vi "Init Sync Box.vi"(8 "error in (no error)":errorcluster, 11 "Channel in":refnum<class "Channel.lvclass">) -> (0 "error out":errorcluster, 3 "Channel out":refnum<class "Channel.lvclass">)   [LabVIEW 2018, in "Channel.lvclass"]
uses:
  Channel.lvclass
  Sync Box/Sync Box.lvclass
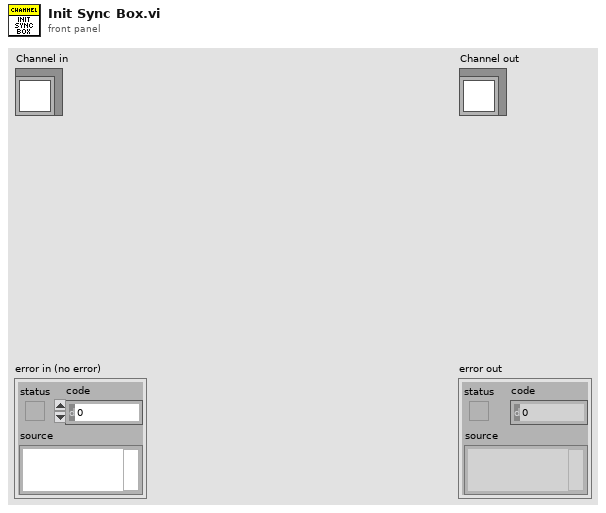
[diagram p1: front panel]
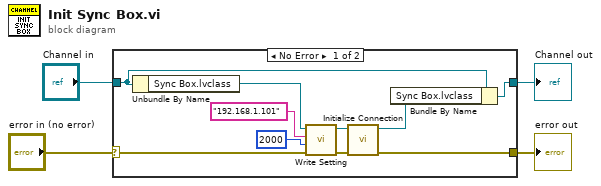
[diagram p0: block diagram]
diagram:
  n1 = case shown="No Error" "error in (no error)" {
    selector: "error in (no error)" -> [w12 w16]
    tunnel: [w6 w16] -> w3
    tunnel: [w5 w15] -> w1
    tunnel: "Channel in" -> [w7 w15]
    frame No Error {
      n2 = Unbundle By Name(w7) -> ("Sync Box.lvclass"=w11:refnum<class "Sync Box.lvclass">)
      n3 = call "Write Setting.vi"("error in (no error)"=w12, "Remote Port"=u32 2000, "Address"="192.168.1.101", "Sync Box in"=w11) -> ("error out"=w13:errorcluster, "Sync Box out"=w14:refnum<class "Sync Box.lvclass">)  [unwired: 6 in]
      n4 = call "Initialize Connection.vi"("error in (no error)"=w13, "Sync Box in"=w14) -> ("error out"=w6:errorcluster, "Sync Box out"=w8:refnum<class "Sync Box.lvclass">)  [unwired: 8 in]
      n5 = Bundle By Name(cluster=w7, "Sync Box.lvclass"=w8) -> (w5:refnum<class "Channel.lvclass">)
    }
    frame Error {
    }
  }
  "error out" <- w3
  "Channel out" <- w1
